vi "autonSample.vi"(0 "Auton Array":dbl[][](array[numeric]), 5 "MeasuredHeading":dbl, 9 "EncoderDistance":dbl) -> (4 "Left Drive":dbl(knob) scale=-1.0..1.0, 6 "Right Drive":dbl(knob) scale=-1.0..1.0, 8 "Ramp ACT motor":dbl, 10 "Turret Rotation":dbl, 13 "Conveyor":dbl, 14 "Harvester":dbl, 15 "Shooter motor output":dbl)   [LabVIEW 2011]
uses:
  Robot Global Data.vi
  <vilib>/addons/control/pid/pid.llb/PID (DBL).vi
  <vilib>/addons/control/pid/NI_PID_pid.lvlib
panel:
  out "Numeric":i16
  out "Tzero":i64
  out "AccumDist":dbl
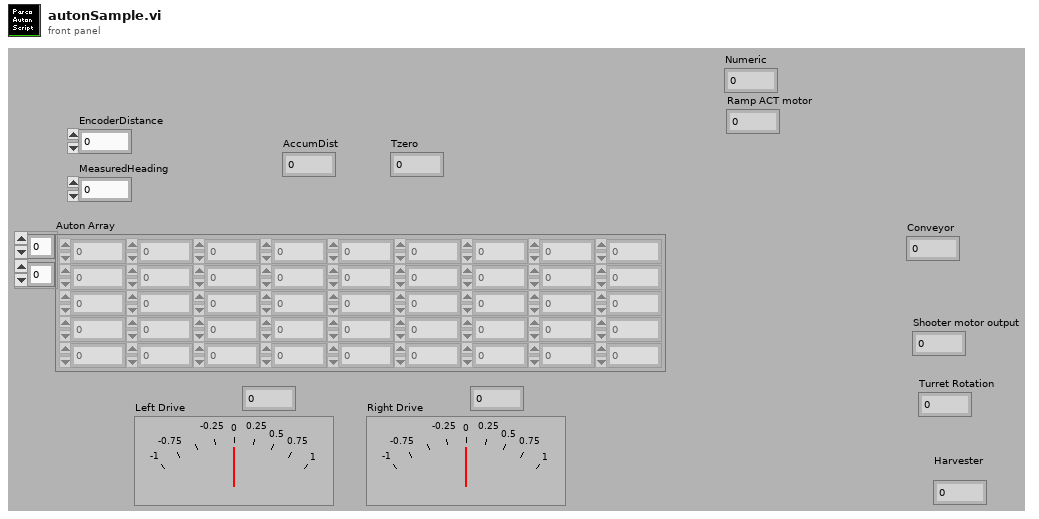
[diagram p1: front panel]
types:
  T1 = cluster{"proportional gain (Kc)":dbl, "integral time (Ti, min)":dbl, "derivative time (Td, min)":dbl}
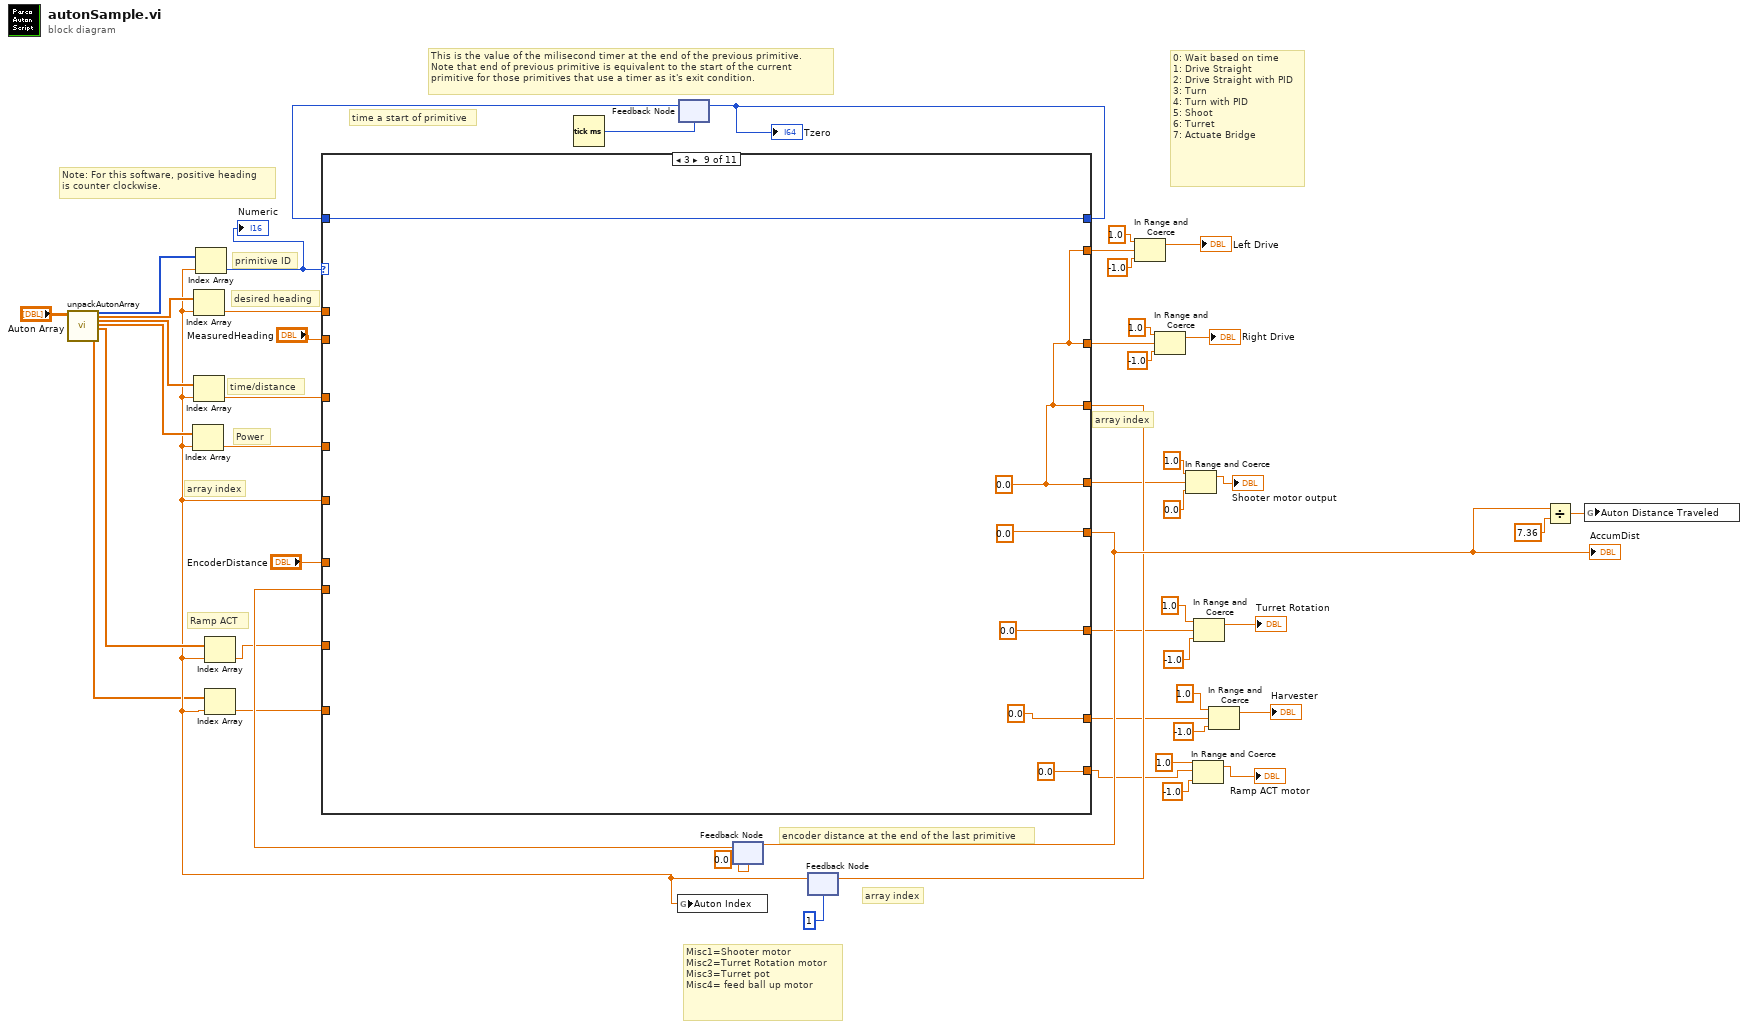
[diagram p0: block diagram]
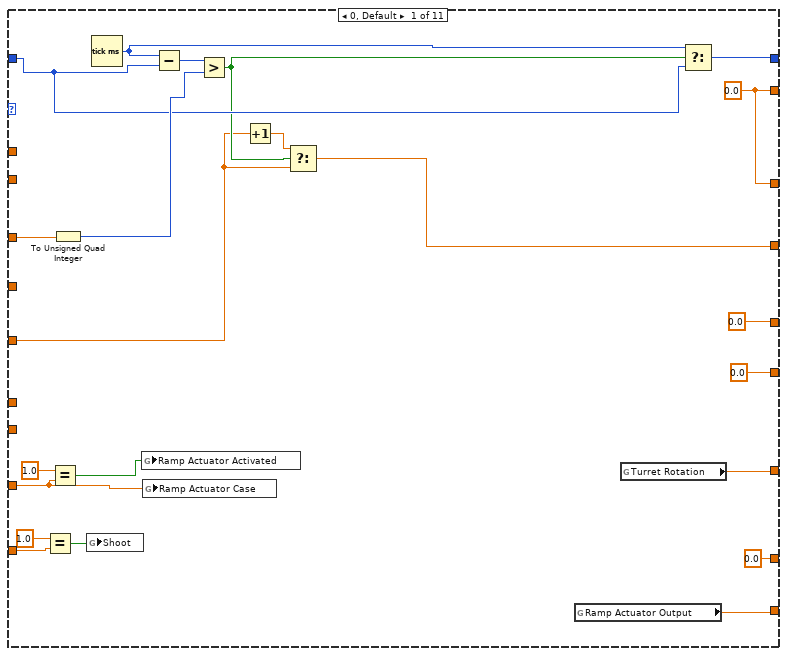
[diagram p2: hidden frame]
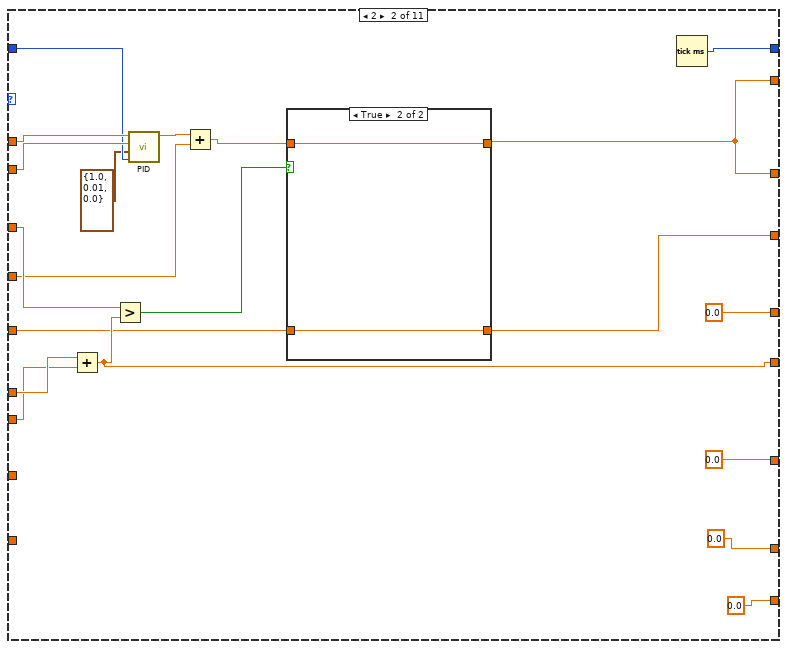
[diagram p3: hidden frame]
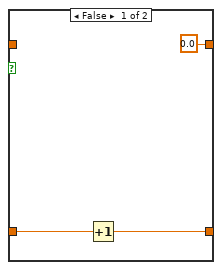
[diagram p4: hidden frame]
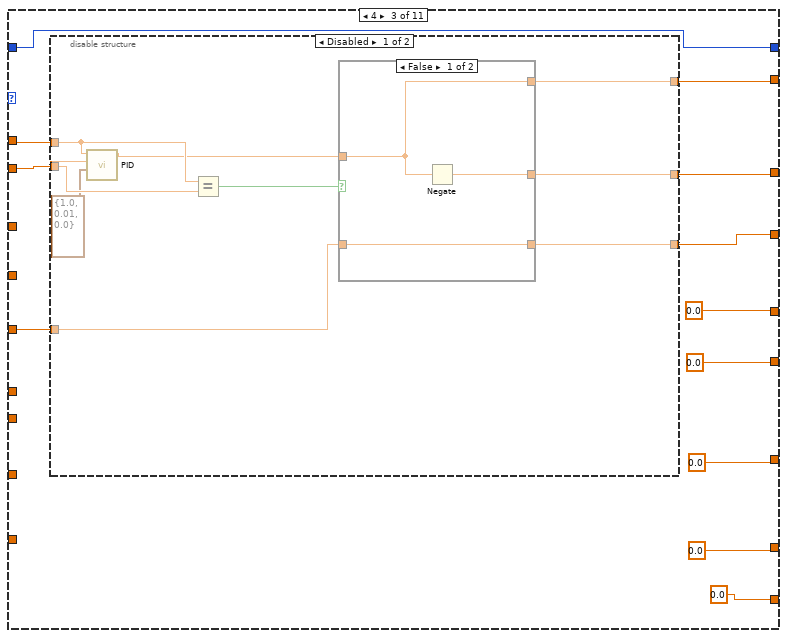
[diagram p5: hidden frame]
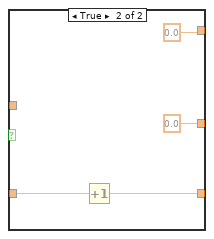
[diagram p6: hidden frame]
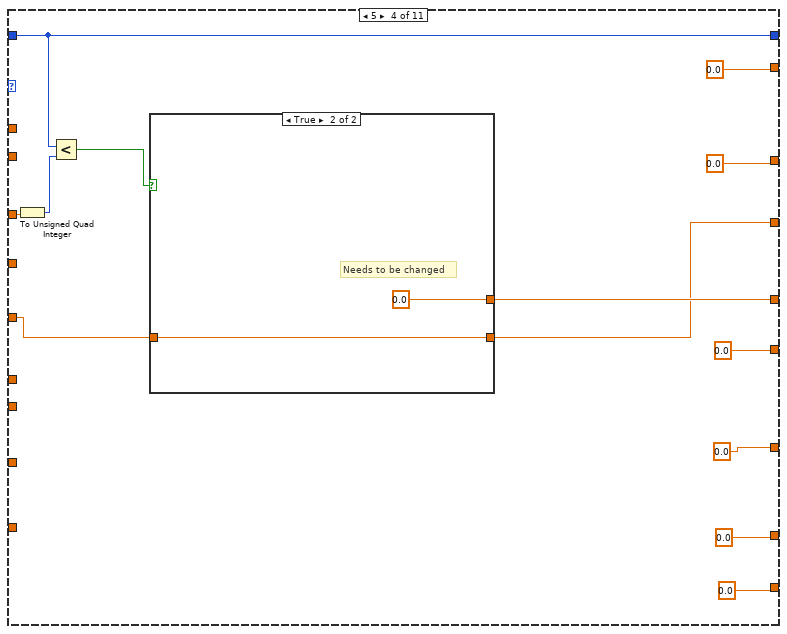
[diagram p8: hidden frame]
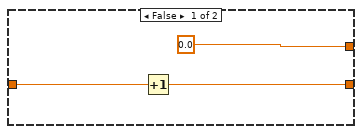
[diagram p9: hidden frame]
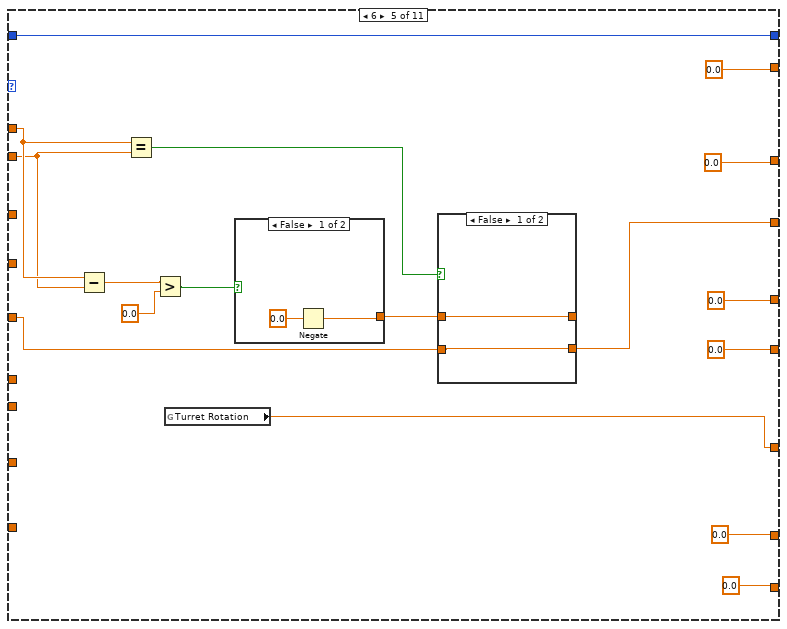
[diagram p10: hidden frame]
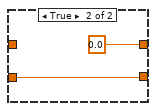
[diagram p11: hidden frame]
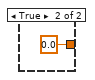
[diagram p12: hidden frame]
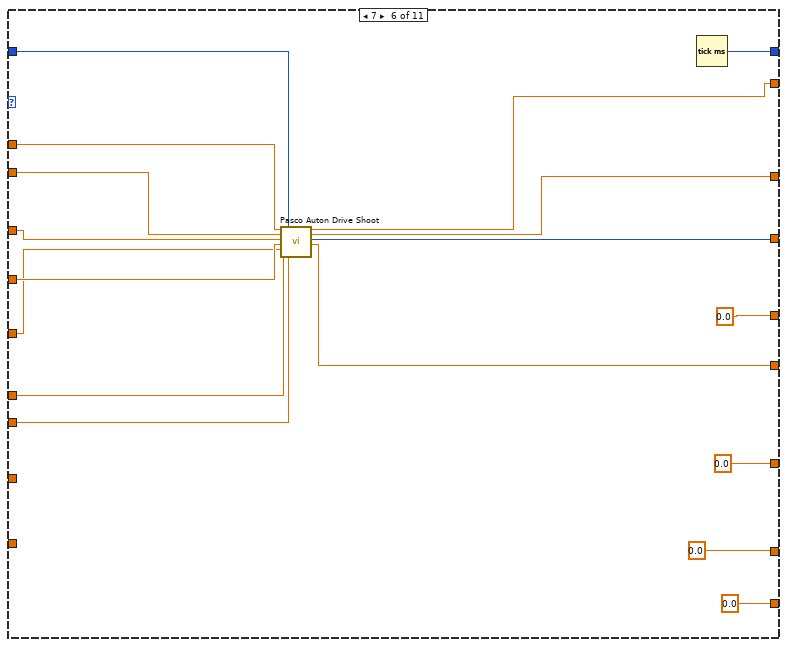
[diagram p13: hidden frame]
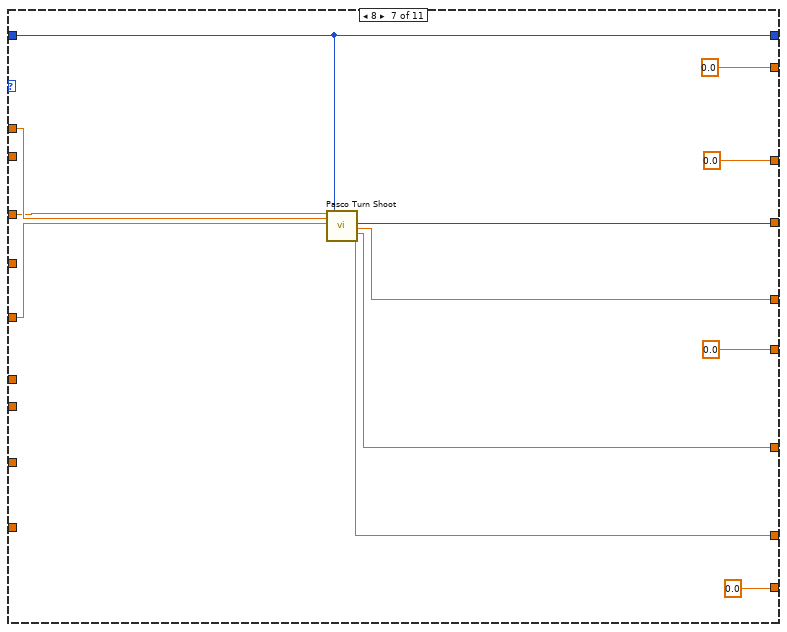
[diagram p14: hidden frame]
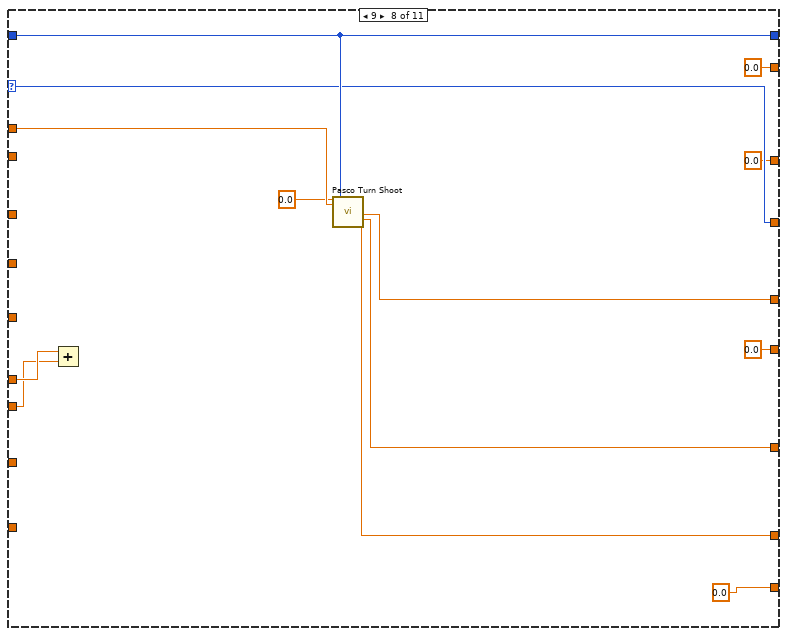
[diagram p15: hidden frame]
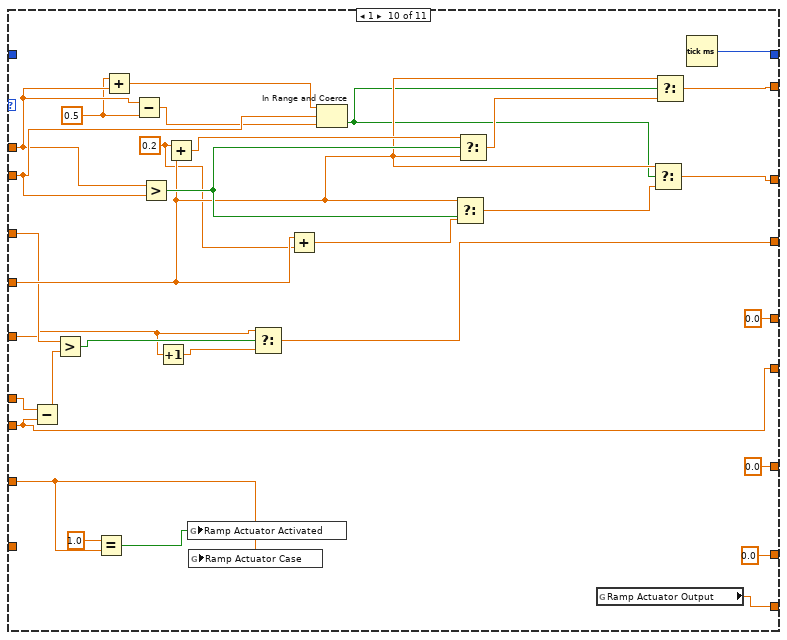
[diagram p16: hidden frame]
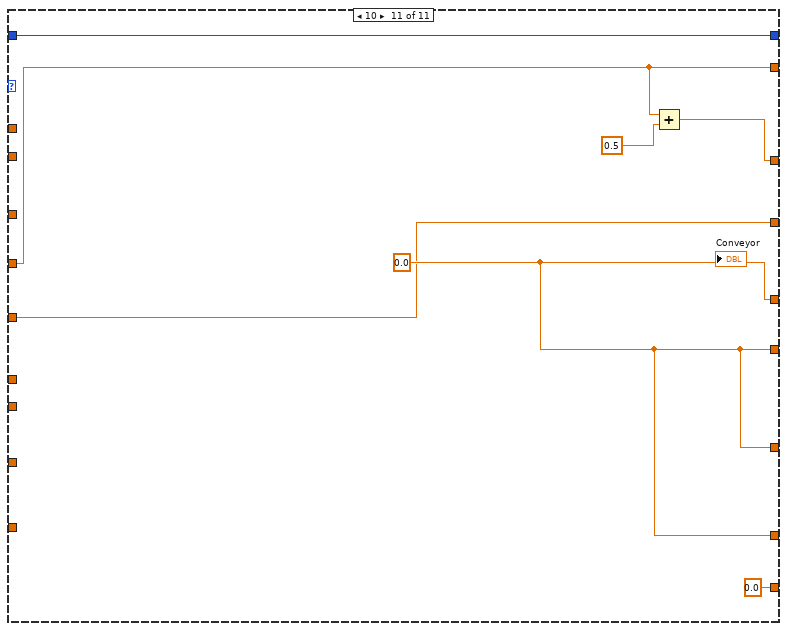
[diagram p17: hidden frame]
diagram:
  # "Ramp ACT"
  # "Misc1=Shooter motor\nMisc2=Turret Rotation motor\nMisc3=Turret pot\nMisc4= feed ball up motor"
  # "0: Wait based on time\n1: Drive Straight\n2: Drive Straight with PID\n3: Turn\n4: Turn with PID\n5: Shoot\n6: Turret\n7: Actuate Bridge"
  # "encoder distance at the end of the last primitive"
  # "Note: For this software, positive heading\nis counter clockwise."
  # "time a start of primitive"
  # "array index"
  # "array index"
  # "This is the value of the milisecond timer at the end of the previous primitive.\nNote that end of previous primitive is equivalent to the start of the current\nprimitive for those primitives that use a timer as it's exit condition."
  # "Power"
  # "array index"
  # "desired heading"
  # "primitive ID"
  # "time/distance"
  n1 = call "unpackAutonArray.vi"("all rows"="Auton Array") -> ("ShootNow"=w2:dbl[], "Primitive"=w49:i16[], "Left Drive"=w32:dbl[], "Right Drive"=w33:dbl[], "Ramp ACT"=w30:dbl[], "Conveyor"=w9:dbl[])  [unwired: 1 in, 20 out]
  n2 = Tick Count (ms)() -> (millisecond timer value=w44:u32)
  n3 = feedback #1(w44) -> (w48:u32)
  n4 = feedback #2(0.0 ("EncoderDistance")) -> (w29:dbl)
  n5 = feedback #3(1) -> (w3:dbl)
  n6 = Index Array(array=w30, index=w3) -> (element=w46:dbl)
  n7 = Index Array(array=w32, index=w3) -> (element=w31:dbl)
  n8 = Index Array(array=w33, index=w3) -> (element=w47:dbl)
  n9 = Index Array(array=w49, index=w3) -> (element=w10:i16)
  "Numeric" <- w10
  n10 = Index Array(array=w9, index=w3) -> (element=w8:dbl)
  n11 = Index Array(array=w2, index=w3) -> (element=w1:dbl)
  n12 = case shown="3" w10 {
    selector: w10 -> [_ _ _ _ _ _ _ w200 _ _ _]
    tunnel: [w60 w85 w103 w133 w156 w169 w193 w200 w210 w226 w252] -> w24
    tunnel: w3 -> [w61 w86 w102 w134 w157 w176 w196 _ _ w224 w252]
    tunnel: [w72 w92 w109 w128 w155 w182 w194 w204 w211 w245 w251] -> w34
    tunnel: w48 -> [w68 w79 w109 w128 w155 w173 w194 w204 w211 _ w251]
    tunnel: w47 -> [w70 w88 _ w138 _ w178 w190 _ _ w228 _]
    tunnel: w31 -> [_ w80 w99 _ w160 w180 w195 w207 _ w238 _]
    tunnel: [w59 w87 w104 0.0 0.0 w172 0.0 0.0 ("Numeric") w210 w229 w249] -> w42
    tunnel: [w59 w87 w105 0.0 0.0 w171 0.0 0.0 ("Right Drive") w210 w230 w248] -> w35
    tunnel: w46 -> [_ w76 _ _ _ w177 _ _ _ w233 w249]
    tunnel: "EncoderDistance" -> [_ w91 _ _ _ w174 _ w209 _ w223 _]
    tunnel: "MeasuredHeading" -> [_ w81 w100 _ w146 w179 _ _ _ w239 _]
    tunnel: [0.0 ("Encoder total") w89 0.0 0.0 0.0 w170 0.0 0.0 ("Encoder total") 0.0 w221 w253] -> w26
    tunnel: w29 -> [_ w90 _ _ _ w175 _ w208 _ w221 _]
    tunnel: [0.0 ("Misc1  OUT") 0.0 0.0 w135 0.0 0.0 ("Misc1  OUT") w192 w206 w210 0.0 ("Misc1  OUT") w253] -> w20
    tunnel: [w54 0.0 0.0 0.0 w145 0.0 ("Misc1  OUT") w191 w205 0.0 0.0 ("Misc2 OUT") w253] -> w16
    tunnel: [0.0 ("Misc4 OUT") 0.0 0.0 0.0 0.0 0.0 w186 w202 0.0 0.0 w253] -> w12
    tunnel: w8 -> [w56 _ _ _ _ _ _ _ _ w219 _]
    tunnel: [w55 0.0 ("Ramp Actuator Output") 0.0 ("Ramp Actuator Output") 0.0 ("Ramp Actuator Output") 0.0 ("Ramp Actuator Output") 0.0 ("Ramp Actuator Output") 0.0 ("Ramp Actuator Output") 0.0 ("Ramp Actuator Output") 0.0 ("Ramp Actuator Output") w216 0.0 ("Ramp Actuator Output")] -> w7
    tunnel: w1 -> [w52 _ _ _ _ _ _ _ _ _ _]
    frame 0, Default {
      w59 = 0.0 ("Numeric")
      n13 = Equal?(x=1.0, y=w52) -> (x = y?=w51:bool)
      n14 = Equal?(x=1.0, y=w56) -> (x = y?=w57:bool)
      n15 = To Unsigned Quad Integer(1:w70) -> (0:w69:u64)
      n16 = global write "Robot Global Data.vi" "Shoot"(w51) -> ()
      n17 = Tick Count (ms)() -> (millisecond timer value=w67:u32)
      n18 = global write "Robot Global Data.vi" "Ramp Actuator Activated"(w57) -> ()
      n19 = global write "Robot Global Data.vi" "Ramp Actuator Case"(w56) -> ()
      n20 = Subtract(x=w67, y=w68) -> (x-y=w71:u32)
      n21 = Greater?(x=w71, y=w69) -> (0:w63:bool)
      n22 = Increment(x=w61) -> (x+1=w62:dbl)
      n23 = Select(t=w62, s=w63, f=w61) -> (s? t:f=w60:dbl)
      n24 = global read "Robot Global Data.vi" "Ramp Actuator Output"() -> (w55:dbl)
      n25 = global read "Robot Global Data.vi" "Turret Rotation"() -> (w54:dbl)
      n26 = Select(t=w67, s=w63, f=w68) -> (s? t:f=w72:u32)
    }
    frame 2 {
      n27 = Add(x=w91, y=w90) -> (x+y=w89:dbl)
      n28 = Greater?(x=w88, y=w89) -> (0:w78:bool)
      n29 = call-poly <vilib>:"PID.vi"("dt (s)"=w79, "PID gains"=T1 {"proportional gain (Kc)"=1.0, "integral time (Ti, min)"=0.01, "derivative time (Td, min)"=0.0}, "process variable"=w81, "setpoint"=w80) -> ("output"=w75:dbl)  [unwired: 6 in, 1 out]
      n30 = Add(x=w75, y=w76) -> (x+y=w74:dbl)
      n31 = case shown="True" w78 {
        tunnel: [0.0 w97] -> w87
        tunnel: w74 -> [_ w97]
        tunnel: w86 -> [w95 w96]
        tunnel: [w94 w96] -> w85
        frame False {
          n32 = Increment(x=w95) -> (x+1=w94:dbl)
        }
        frame True {
        }
      }
      n33 = Tick Count (ms)() -> (millisecond timer value=w92:u32)
    }
    frame 4 {
      n34 = disable-structure shown="Disabled" {
        disable-tunnel: [w118 _] -> w105
        disable-tunnel: [w117 _] -> w104
        disable-tunnel: [w116 _] -> w103
        disable-tunnel: w102 -> [w115 _]
        disable-tunnel: w100 -> [w113 _]
        disable-tunnel: w99 -> [w112 _]
        frame Disabled {
          n35 = call-poly <vilib>:"PID.vi"("PID gains"=T1 {"proportional gain (Kc)"=1.0, "integral time (Ti, min)"=0.01, "derivative time (Td, min)"=0.0}, "process variable"=w113, "setpoint"=w112) -> ("output"=w111:dbl)  [unwired: 7 in, 1 out]
          n36 = Equal?(x=w112, y=w113) -> (x = y?=w114:bool)
          n37 = case shown="False" w114 {
            tunnel: w111 -> [w120 _]
            tunnel: [w121 0.0] -> w118
            tunnel: [w120 0.0] -> w117
            tunnel: [w119 w124] -> w116
            tunnel: w115 -> [w119 w125]
            frame False {
              n38 = Negate(x=w120) -> (-x=w121:dbl)
            }
            frame True {
              n39 = Increment(x=w125) -> (x+1=w124:dbl)
            }
          }
        }
        frame Enabled {
        }
      }
    }
    frame 5 {
      n40 = To Unsigned Quad Integer(1:w138) -> (0:w136:u64)
      n41 = Less?(x=w128, y=w136) -> (x < y?=w137:bool)
      n42 = case shown="True" w137 {
        tunnel: [0.0 0.0] -> w135
        tunnel: w134 -> [w140 w143]
        tunnel: [w139 w143] -> w133
        frame False {
          n43 = Increment(x=w140) -> (x+1=w139:dbl)
        }
        frame True {
          # "Needs to be changed"
        }
      }
    }
    frame 6 {
      n44 = Subtract(x=w160, y=w146) -> (x-y=w148:dbl)
      n45 = Equal?(x=w160, y=w146) -> (x = y?=w159:bool)
      n46 = Greater?(x=w148, y=0.0) -> (0:w149:bool)
      n47 = global read "Robot Global Data.vi" "Turret Rotation"() -> (w145:dbl)
      n48 = case shown="False" w149 {
        tunnel: [w166 0.0] -> w158
        frame False {
          n49 = Negate(x=0.0) -> (-x=w166:dbl)
        }
        frame True {
        }
      }
      n50 = case shown="False" w159 {
        tunnel: [w162 0.0] -> _
        tunnel: w158 -> [w162 _]
        tunnel: w157 -> [w161 w164]
        tunnel: [w161 w164] -> w156
        frame False {
        }
        frame True {
        }
      }
    }
    frame 7 {
      n51 = call "Pasco Auton Drive Shoot.vi"("Desired Heading"=w180, "Actual Heading"=w179, "time/distance"=w178, "Power"=w177, "Array"=w176, "Encoder total"=w174, "Time"=w173, "Encoder Return"=w175) -> ("Left Drive"=w172:dbl, "Right Drive"=w171:dbl, "Array Out"=w169:i32, "Encoder total"=w170:dbl)  [unwired: 8 in]
      n52 = Tick Count (ms)() -> (millisecond timer value=w182:u32)
    }
    frame 8 {
      n53 = call "Pasco Turn Shoot.vi"("time/distance"=w190, "desired heading"=w195, "array index"=w196, "primitive time"=w194) -> ("array index"=w193:i32, "Misc1  OUT"=w192:dbl, "Misc2 OUT"=w191:dbl, "Misc4 OUT"=w186:dbl)  [unwired: 12 in]
    }
    frame 9 {
      n54 = Add(x=w209, y=w208) -> ()  [unwired: 1 out]
      n55 = call "Pasco Turn Shoot.vi"("time/distance"=0.0, "desired heading"=w207, "primitive time"=w204) -> ("Misc1  OUT"=w206:dbl, "Misc2 OUT"=w205:dbl, "Misc4 OUT"=w202:dbl)  [unwired: 13 in, 1 out]
    }
    frame 3 {
      w210 = 0.0
    }
    frame 1 {
      w237 = 0.5 ("x")
      w220 = 0.2 ("x")
      n56 = Subtract(x=w223, y=w221) -> (x-y=w222:dbl)
      n57 = Greater?(x=w228, y=w222) -> (0:w227:bool)
      n58 = Equal?(x=1.0, y=w219) -> (x = y?=w217:bool)
      n59 = Add(x=w237, y=w238) -> (x+y=w235:dbl)
      n60 = Subtract(x=w238, y=w237) -> (x-y=w236:dbl)
      n61 = Greater?(x=w238, y=w239) -> (0:w241:bool)
      n62 = Increment(x=w224) -> (x+1=w225:dbl)
      n63 = Add(x=w220, y=w233) -> (x+y=w242:dbl)
      n64 = global write "Robot Global Data.vi" "Ramp Actuator Activated"(w217) -> ()
      n65 = global write "Robot Global Data.vi" "Ramp Actuator Case"(w219) -> ()
      n66 = Select(t=w224, s=w227, f=w225) -> (s? t:f=w226:dbl)
      n67 = Add(x=w233, y=w220) -> (x+y=w240:dbl)
      n68 = In Range and Coerce(upper limit=w235, x=w239, lower limit=w236) -> (In Range?=w232:bool)  [unwired: 1 out]
      n69 = Select(t=w233, s=w241, f=w240) -> (s? t:f=w231:dbl)
      n70 = Select(t=w242, s=w241, f=w233) -> (s? t:f=w234:dbl)
      n71 = global read "Robot Global Data.vi" "Ramp Actuator Output"() -> (w216:dbl)
      n72 = Select(t=w233, s=w232, f=w231) -> (s? t:f=w230:dbl)
      n73 = Select(t=w233, s=w232, f=w234) -> (s? t:f=w229:dbl)
      n74 = Tick Count (ms)() -> (millisecond timer value=w245:u32)
    }
    frame 10 {
      w253 = 0.0
      n75 = Add(x=w249, y=0.5 ("x+y")) -> (x+y=w248:dbl)
    }
  }
  "AccumDist" <- w26
  "Tzero" <- w34
  n76 = global write "Robot Global Data.vi" "Auton Index"(w3) -> ()
  n77 = feedback-in #1(w34) -> ()
  n78 = feedback-in #2(w26) -> ()
  n79 = feedback-in #3(w24) -> ()
  n80 = In Range and Coerce(upper limit=1.0, x=w42, lower limit=-1.0) -> (coerced(x)=→"Left Drive":dbl)  [unwired: 1 out]
  n81 = In Range and Coerce(upper limit=1.0, x=w35, lower limit=-1.0) -> (coerced(x)=→"Right Drive":dbl)  [unwired: 1 out]
  n82 = In Range and Coerce(upper limit=1.0, x=w20, lower limit=0.0) -> (coerced(x)=→"Shooter motor output":dbl)  [unwired: 1 out]
  n83 = In Range and Coerce(upper limit=1.0, x=w7, lower limit=-1.0) -> (coerced(x)=→"Ramp ACT motor":dbl)  [unwired: 1 out]
  n84 = In Range and Coerce(upper limit=1.0, x=w16, lower limit=-1.0) -> (coerced(x)=→"Turret Rotation":dbl)  [unwired: 1 out]
  n85 = In Range and Coerce(upper limit=1.0, x=w12, lower limit=-1.0) -> (coerced(x)=→"Harvester":dbl)  [unwired: 1 out]
  n86 = Divide(x=w26, y=7.36) -> (x/y=w11:dbl)
  n87 = global write "Robot Global Data.vi" "Auton Distance Traveled"(w11) -> ()
